vi "HMI Project.vi"() -> ()   [LabVIEW 2017]
uses:
  <vilib>/Instr/_visa.llb/VISA Configure Serial Port (Instr).vi
panel:
  in  "Alamat IP RTU 3 (192.168.4.1)":string
  out "?":dbl(slide) scale=0.0..125.0
  out "?":dbl(knob) scale=0.0..1200.0
  out "Grafik Tekanan RTU 3 (kPa)":dbl(graph)
  out "Grafik Jarak RTU 3 (meter)":dbl(graph)
  out "Jarak RTU 3 (meter)":dbl
  out "Tekanan RTU 3 (kPa)":dbl
  out "Longitude 2":dbl
  out "Latitude":dbl
  out "?":string
  out "?":dbl(slide) scale=0.0..125.0
  out "?":dbl(knob) scale=0.0..1200.0
  out "Grafik Tekanan RTU 1 (kPa)":dbl(graph)
  out "Grafik Jarak RTU 1 (meter)":dbl(graph)
  out "?":dbl(slide) scale=0.0..125.0
  out "?":dbl(knob) scale=0.0..1200.0
  out "Grafik Tekanan RTU 2 (kPa)":dbl(graph)
  out "Grafik Jarak RTU 2 (meter)":dbl(graph)
  out "Jarak RTU 2 (meter)":dbl
  out "Tekanan RTU 2 (kPa)":dbl
  out "Longitude":dbl
  out "Latitude":dbl
  in  "Pilih Port (COM 4)":refnum<visa-resource-name>
  out "Jarak RTU 1 (meter)":dbl
  out "Tekanan RTU 1 (kPa)":dbl
  out "Longitude":dbl
  out "Latitude":dbl
  in  "?":bool
  out "?":string
  in  "Alamat IP RTU 1 (192.168.2.113)":string
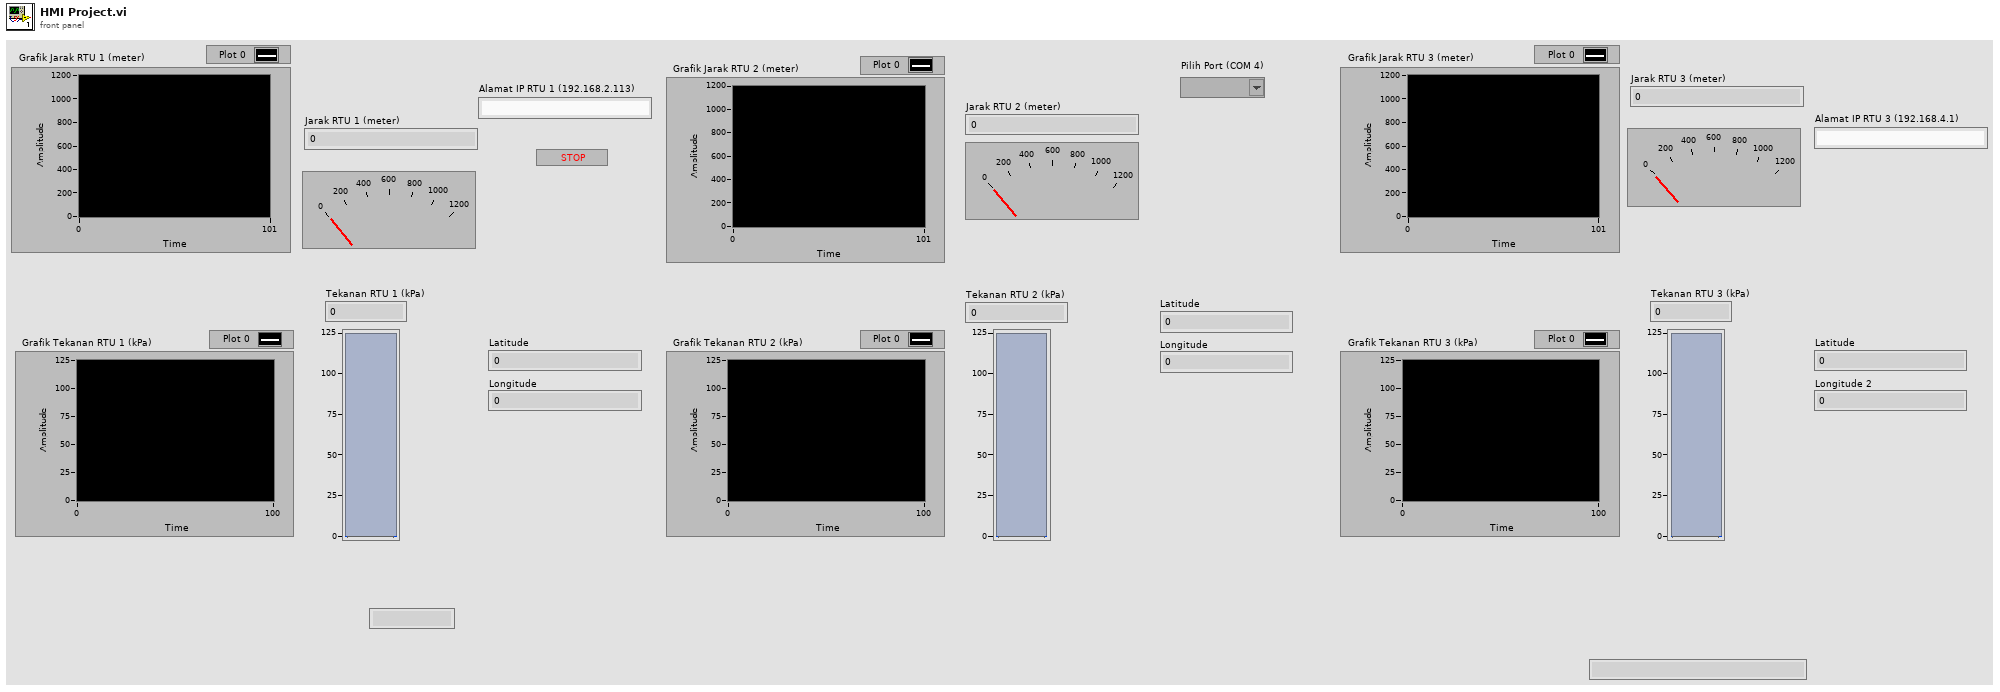
[diagram p1: front panel]
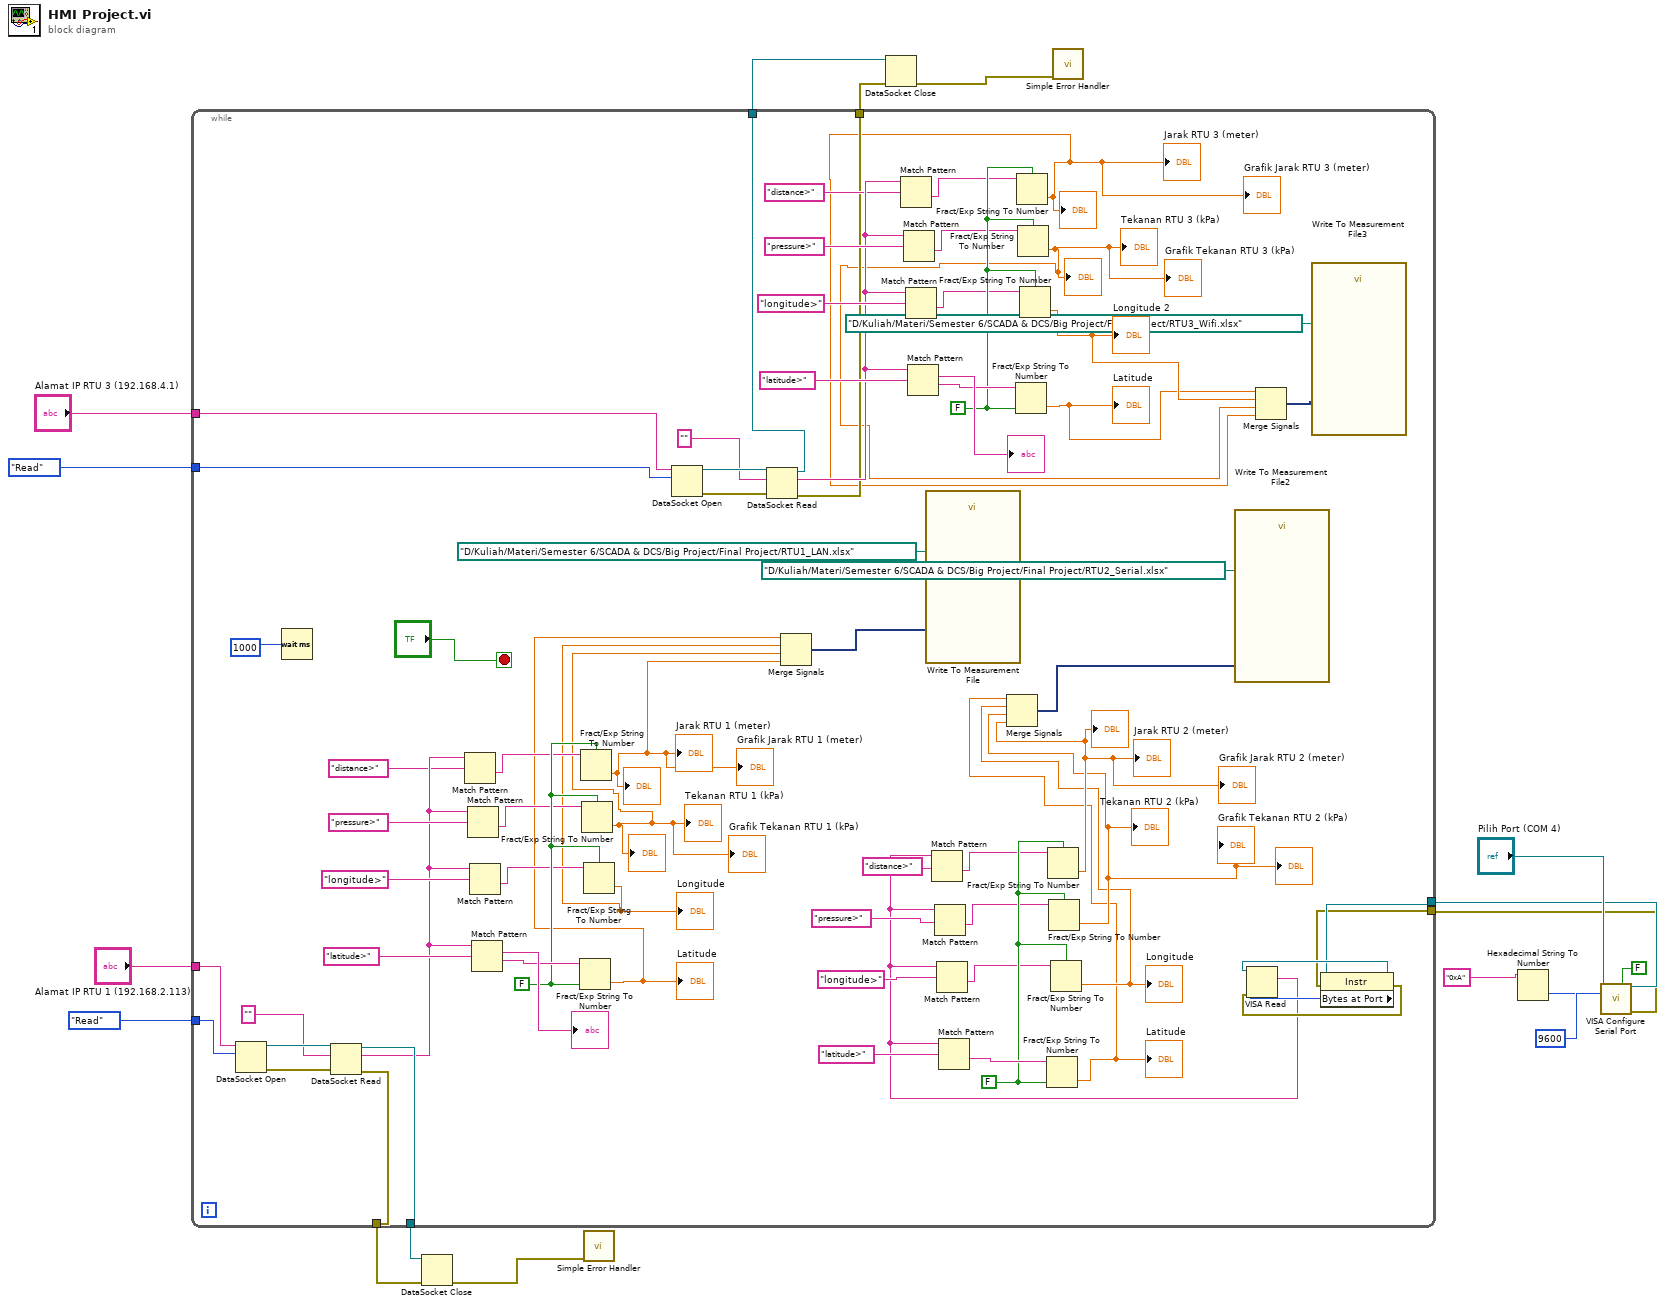
[diagram p0: block diagram]
diagram:
  n1 = Hexadecimal String To Number(string="0xA") -> (number=w7:u32)  [unwired: 2 in, 1 out]
  n2 = call-poly "VISA Configure Serial Port"("VISA resource name"="Pilih Port (COM 4)", "termination char\n(0xA = '\\n' = LF)"=w7, "Enable Termination\nChar (T)"=FALSE ("Enable Termination\nChar (T)"), "baud rate (9600)"=u32 9600) -> ("VISA resource name out"=w10:refnum<visa-resource-name>, "error out"=w9:errorcluster)  [unwired: 10 in]
  n3 = while {
    tunnel: [w84] -> w16
    tunnel: [w82] -> w15
    tunnel: "Alamat IP RTU 1 (192.168.2.113)" -> [w80]
    tunnel: enum16{"Read"}."Read" -> [w79]
    tunnel: w10 -> [w66]
    tunnel: w9 -> [w65]
    tunnel: "Alamat IP RTU 3 (192.168.4.1)" -> [w39]
    tunnel: enum16{"Read"}."Read" -> [w38]
    tunnel: [w37] -> w2
    tunnel: [w36] -> w1
    stop <- "?" stop-if-true
    w44 = FALSE
    w59 = FALSE
    w73 = FALSE
    n4 = DataSocket Open(10:w79, 11:w80) -> (0:w85:errorcluster, 3:w88:refnum<k13>)  [unwired: 2 in]
    n5 = Wait (ms)(milliseconds to wait=1000) -> ()  [unwired: 1 out]
    n6 = DataSocket Read(8:w85, 10:"", 11:w88) -> (0:w84:errorcluster, 2:w74:string, 3:w82:refnum<k13>)  [unwired: 2 in, 4 out]
    n7 = Match Pattern(string=w74, regular expression="distance>") -> (after substring=w70:string)  [unwired: 1 in, 3 out]
    n8 = Match Pattern(string=w74, regular expression="pressure>") -> (after substring=w71:string)  [unwired: 1 in, 3 out]
    n9 = Match Pattern(string=w74, regular expression="longitude>") -> (after substring=w72:string)  [unwired: 1 in, 3 out]
    n10 = Match Pattern(string=w74, regular expression="latitude>") -> (match substring=→"?":string, after substring=w77:string)  [unwired: 1 in, 2 out]
    n11 = Fract/Exp String To Number(use system decimal point (T)=w73, string=w77) -> (number=w25:dbl)  [unwired: 2 in, 1 out]
    "Latitude" <- w25
    n12 = Fract/Exp String To Number(use system decimal point (T)=w73, string=w70) -> (number=w28:dbl)  [unwired: 2 in, 1 out]
    "Jarak RTU 1 (meter)" <- w28
    "Grafik Jarak RTU 1 (meter)" <- w28
    "?" <- w28
    n13 = Fract/Exp String To Number(use system decimal point (T)=w73, string=w71) -> (number=w27:dbl)  [unwired: 2 in, 1 out]
    "Tekanan RTU 1 (kPa)" <- w27
    "Grafik Tekanan RTU 1 (kPa)" <- w27
    "?" <- w27
    n14 = Fract/Exp String To Number(use system decimal point (T)=w73, string=w72) -> (number=w26:dbl)  [unwired: 2 in, 1 out]
    "Longitude" <- w26
    n15 = DataSocket Open(10:w38, 11:w39) -> (0:w50:errorcluster, 3:w53:refnum<k13>)  [unwired: 2 in]
    n16 = DataSocket Read(8:w50, 10:"", 11:w53) -> (0:w36:errorcluster, 2:w45:string, 3:w37:refnum<k13>)  [unwired: 2 in, 4 out]
    n17 = Merge Signals(w25, w26, w27, w28) -> (w29:dynamicdata)
    n18 = Match Pattern(string=w45, regular expression="distance>") -> (after substring=w41:string)  [unwired: 1 in, 3 out]
    n19 = Match Pattern(string=w45, regular expression="pressure>") -> (after substring=w42:string)  [unwired: 1 in, 3 out]
    n20 = Match Pattern(string=w45, regular expression="longitude>") -> (after substring=w43:string)  [unwired: 1 in, 3 out]
    n21 = Match Pattern(string=w45, regular expression="latitude>") -> (match substring=→"?":string, after substring=w48:string)  [unwired: 1 in, 2 out]
    n22 = call "Write To Measurement File"("Signals"=w29, "Filename"=path "D:/Kuliah/Materi/Semester 6/SCADA & DCS/Big Project/Final Project/RTU1_LAN.xlsx") -> ()  [unwired: 15 in, 3 out]
    n23 = Fract/Exp String To Number(use system decimal point (T)=w44, string=w48) -> (number=w18:dbl)  [unwired: 2 in, 1 out]
    "Latitude" <- w18
    n24 = Fract/Exp String To Number(use system decimal point (T)=w44, string=w41) -> (number=w21:dbl)  [unwired: 2 in, 1 out]
    "Jarak RTU 3 (meter)" <- w21
    "Grafik Jarak RTU 3 (meter)" <- w21
    "?" <- w21
    n25 = Fract/Exp String To Number(use system decimal point (T)=w44, string=w42) -> (number=w20:dbl)  [unwired: 2 in, 1 out]
    "Tekanan RTU 3 (kPa)" <- w20
    "Grafik Tekanan RTU 3 (kPa)" <- w20
    "?" <- w20
    n26 = Fract/Exp String To Number(use system decimal point (T)=w44, string=w43) -> (number=w19:dbl)  [unwired: 2 in, 1 out]
    "Longitude 2" <- w19
    n27 = Merge Signals(w18, w19, w20, w21) -> (w22:dynamicdata)
    n28 = call "Write To Measurement File3"("Signals"=w22, "Filename"=path "D:/Kuliah/Materi/Semester 6/SCADA & DCS/Big Project/Final Project/RTU3_Wifi.xlsx") -> ()  [unwired: 15 in, 3 out]
    n29 = property class="Instr"(reference=w66, error in=w65) -> (reference out=w69:refnum<visa-resource-name>, error out=w67:errorcluster, "Bytes at Port"=w68:u32)
    n30 = VISA Read(VISA resource name=w69, byte count=w68, error in (no error)=w67) -> (read buffer=w55:string)  [unwired: 3 out]
    n31 = Match Pattern(string=w55, regular expression="distance>") -> (after substring=w56:string)  [unwired: 1 in, 3 out]
    n32 = Match Pattern(string=w55, regular expression="pressure>") -> (after substring=w57:string)  [unwired: 1 in, 3 out]
    n33 = Match Pattern(string=w55, regular expression="longitude>") -> (after substring=w58:string)  [unwired: 1 in, 3 out]
    n34 = Match Pattern(string=w55, regular expression="latitude>") -> (after substring=w63:string)  [unwired: 1 in, 3 out]
    n35 = Fract/Exp String To Number(use system decimal point (T)=w59, string=w63) -> (number=w31:dbl)  [unwired: 2 in, 1 out]
    "Latitude" <- w31
    n36 = Fract/Exp String To Number(use system decimal point (T)=w59, string=w56) -> (number=w34:dbl)  [unwired: 2 in, 1 out]
    "Jarak RTU 2 (meter)" <- w34
    "Grafik Jarak RTU 2 (meter)" <- w34
    "?" <- w34
    n37 = Fract/Exp String To Number(use system decimal point (T)=w59, string=w57) -> (number=w33:dbl)  [unwired: 2 in, 1 out]
    "Tekanan RTU 2 (kPa)" <- w33
    "Grafik Tekanan RTU 2 (kPa)" <- w33
    "?" <- w33
    n38 = Fract/Exp String To Number(use system decimal point (T)=w59, string=w58) -> (number=w32:dbl)  [unwired: 2 in, 1 out]
    "Longitude" <- w32
    n39 = Merge Signals(w31, w32, w33, w34) -> (w35:dynamicdata)
    n40 = call "Write To Measurement File2"("Signals"=w35, "Filename"=path "D:/Kuliah/Materi/Semester 6/SCADA & DCS/Big Project/Final Project/RTU2_Serial.xlsx") -> ()  [unwired: 15 in, 3 out]
  }
  n41 = DataSocket Close(8:w16, 11:w15) -> (0:w17:errorcluster)  [unwired: 1 in, 1 out]
  n42 = call <vilib>:"Simple Error Handler.vi"("error in (no error)"=w17) -> ()  [unwired: 4 in, 5 out]
  n43 = DataSocket Close(8:w1, 11:w2) -> (0:w3:errorcluster)  [unwired: 1 in, 1 out]
  n44 = call <vilib>:"Simple Error Handler.vi"("error in (no error)"=w3) -> ()  [unwired: 4 in, 5 out]
